vi "AtDome_acceptCommand_disable.vi"(8 "error in (no error)":errorcluster, 11 "command_disable_Ctl":T1={"device"="", "property"="                                ", "action"="                                ", "itemValue"="                                ", "value"=FALSE}) -> (0 "error out":errorcluster, 2 "function return":i32, 3 "command_disable_Ctl out":T1={"device"="", "property"="                                ", "action"="                                ", "itemValue"="                                ", "value"=FALSE})   [LabVIEW 2016, in "SALLV_AtDome.lvlib"]
doc: "int AtDome_shm_acceptCommand_disableLV(AtDome_command_disableLV *command_disable_Ctl );"
uses:
  SALLV_AtDome.lvlib
  DataTypes/command_disable.ctl
  SALLV_AtDome.so
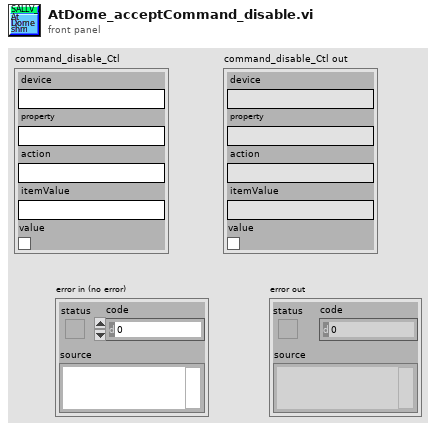
[diagram p1: front panel]
types:
  T1 = typedef "SALLV_AtDome.lvlib/command_disable.ctl" = cluster{"device":string, "property":string, "action":string, "itemValue":string, "value":bool}
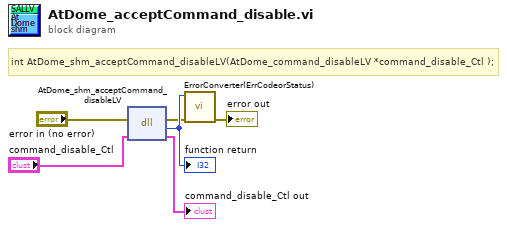
[diagram p0: block diagram]
diagram:
  # "int AtDome_shm_acceptCommand_disableLV(AtDome_command_disableLV *command_disable_Ctl );"
  n1 = dll-call lib="home/andres/Desktop/SAL_AtDome/SALLV_AtDome.*" fn="AtDome_shm_acceptCommand_disableLV"(error in="error in (no error)", "command_disable_Ctl"="command_disable_Ctl") -> (error out=w2:errorcluster, w6:i32, "command_disable_Ctl"=→"command_disable_Ctl out":T1)  [unwired: 2 in, 1 out]
  "function return" <- w6
  n2 = call "ErrorConverter(ErrCodeorStatus).vi"("error in (no error)"=w2, "error code"=w6) -> ("error out"=→"error out":errorcluster)  [unwired: 9 in]
